vi "SeCrTs-Datalog Display NS creater.vi"(9 "Data FIFO Ref":T1) -> ()   [LabVIEW 2022 SP3]
uses:
  RT Controls/SeCrTs-Data FIFO.ctl
  RT Controls/SeCrTs-DiplayPC comm ctrl.ctl
  <vilib>/dex/Stream Element Allocation Mode.ctl
  SeCrTs-RT_Global_R.vi
  <resource>/objmgr/ni.dex.rc
panel:
  out "Numeric":i32
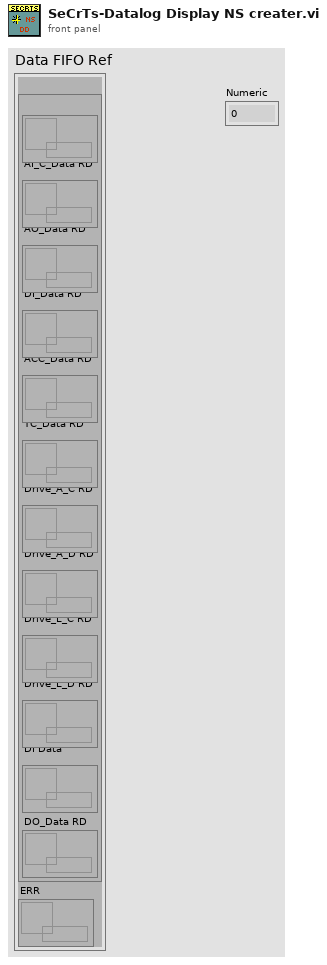
[diagram p1: front panel]
types:
  T1 = typedef "SeCrTs-Data FIFO.ctl" = cluster{"RD":cluster{"AI_V_Data RD":refnum<queue>, "AI_C_Data RD":refnum<queue>, "AO_Data RD":refnum<queue>, "DI_Data RD":refnum<queue>, "ACC_Data RD":refnum<queue>, "TC_Data RD":refnum<queue>, "Drive_A_C RD":refnum<queue>, "Drive_A_D RD":refnum<queue>, "Drive_L_C RD":refnum<queue>, "Drive_L_D RD":refnum<queue>, "DI Data":refnum<queue>, "DO_Data RD":refnum<queue>}, "ERR":refnum<queue>}
  T2 = typedef "SeCrTs-DiplayPC comm ctrl.ctl" = enum16{"Initialize", "Listen for UI Writer", "Send RT Data"}
  T3 = typedef "Stream Element Allocation Mode.ctl" = u32
  T4 = cluster{"Start DAQ":bool, "Stop DAQ":bool, "RT Stop":bool, "RT Exit":bool, "Start Seq":bool}
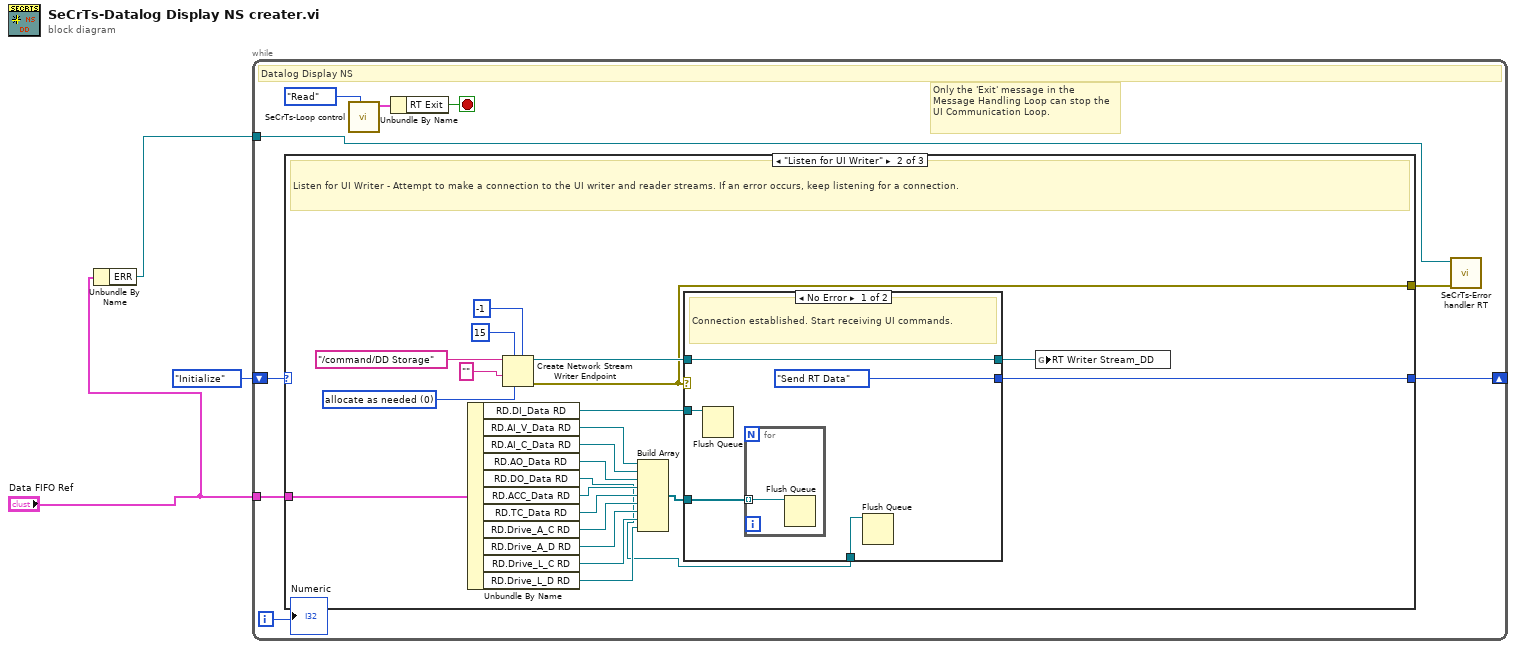
[diagram p0: block diagram]
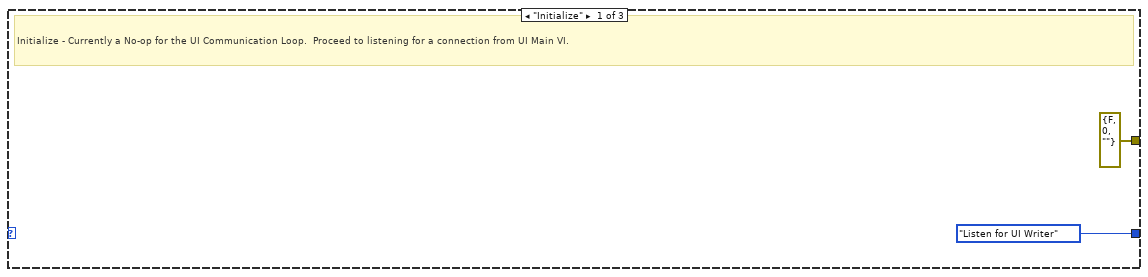
[diagram p2: hidden frame]
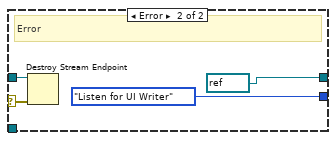
[diagram p3: hidden frame]
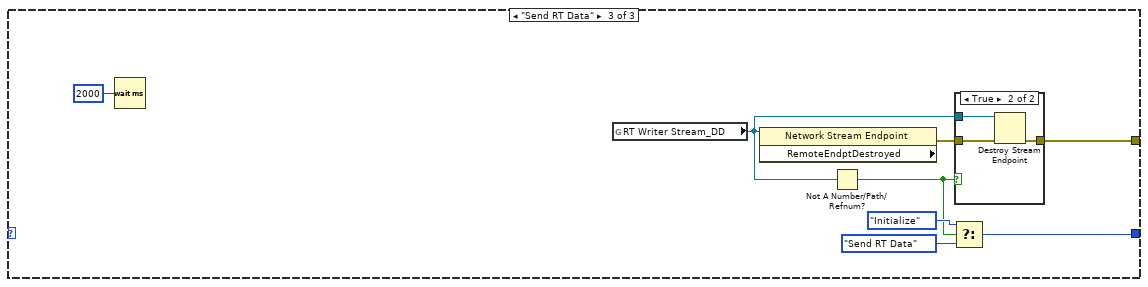
[diagram p4: hidden frame]
diagram:
  n1 = Unbundle By Name("Data FIFO Ref") -> ("ERR"=w1:refnum<queue>)
  n2 = while {
    shift-right: [w12] -> _
    shift-left: SeCrTs-DiplayPC_comm_ctrl."Initialize" -> [w11]
    tunnel: "Data FIFO Ref" -> [w10]
    tunnel: w1 -> [w6]
    i -> [w4]
    stop <- w7 stop-if-true
    # "Only the 'Exit' message in the  Message Handling Loop can stop the UI Communication Loop."
    # "Datalog Display NS"
    n3 = case shown="\"Listen for UI Writer\"" w11 {
      tunnel: [errorcluster {"status"=FALSE, "code"=0, "source"=""} ("error IO") w35 w47] -> w5
      tunnel: [SeCrTs-DiplayPC_comm_ctrl."Listen for UI Writer" w34 w53] -> w12
      tunnel: w10 -> [_ w31 _]
      frame "Initialize" {
        # "Initialize - Currently a No-op for the UI Communication Loop.  Proceed to listening for a connection from UI Main VI."
      }
      frame "Listen for UI Writer" {
        w16 = T3 0 items=["allocate as needed", "pre-allocate"] ("element allocation mode")
        # "Listen for UI Writer - Attempt to make a connection to the UI writer and reader streams. If an error occurs, keep listening for a connection."
        n4 = Unbundle By Name(w31) -> ("RD.DI_Data RD"=w18:refnum<queue>, "RD.AI_V_Data RD"=w28:refnum<queue>, "RD.AI_C_Data RD"=w27:refnum<queue>, "RD.AO_Data RD"=w26:refnum<queue>, "RD.DO_Data RD"=w15:refnum<queue>, "RD.ACC_Data RD"=w25:refnum<queue>, "RD.TC_Data RD"=w24:refnum<queue>, "RD.Drive_A_C RD"=w23:refnum<queue>, "RD.Drive_A_D RD"=w22:refnum<queue>, "RD.Drive_L_C RD"=w21:refnum<queue>, "RD.Drive_L_D RD"=w20:refnum<queue>)
        n5 = Create Network Stream Writer Endpoint(5:-1 ("timeout in ms (-1)"), 6:w16, 7:15 ("writer buffer size"), 9:"" ("reader url"), 11:"/command/DD Storage" ("reader url")) -> (0:w35:errorcluster, 3:w36:refnum<k21>)  [unwired: 2 in]
        n6 = Build Array(w28, w27, w26, w25, w24, w23, w22, w21, w20) -> (w19:refnum<queue>[])
        n7 = case shown="No Error" w35 {
          selector: w35 -> [_ w44]
          tunnel: w36 -> [w40 w46]
          tunnel: [SeCrTs-DiplayPC_comm_ctrl."Send RT Data" SeCrTs-DiplayPC_comm_ctrl."Listen for UI Writer"] -> w34
          tunnel: [w40 refnum<k21> refnum ("reader url")] -> w29
          tunnel: w19 -> [w39 _]
          tunnel: w18 -> [w38 _]
          tunnel: w15 -> [w37 _]
          frame No Error {
            # "Connection established. Start receiving UI commands."
            n8 = Flush Queue(queue=w38) -> ()  [unwired: 1 in, 3 out]
            n9 = for {
              tunnel: w39 -> [w42] mode=indexing
              n10 = Flush Queue(queue=w42) -> ()  [unwired: 1 in, 3 out]
            }
            n11 = Flush Queue(queue=w37) -> ()  [unwired: 1 in, 3 out]
          }
          frame Error {
            # "Error"
            n12 = Destroy Stream Endpoint(8:w44, 11:w46) -> ()  [unwired: 1 out]
          }
        }
        n13 = global write "SeCrTs-RT_Global_R.vi" "RT Writer Stream_DD"(w29) -> ()
      }
      frame "Send RT Data" {
        n14 = Wait (ms)(milliseconds to wait=u32 2000) -> ()  [unwired: 1 out]
        n15 = global read "SeCrTs-RT_Global_R.vi" "RT Writer Stream_DD"() -> (w49:refnum<k21>)
        n16 = property class="Network Stream Endpoint" props=["RemoteEndptDestroyed"](reference=w49) -> (error out=w48:errorcluster)  [unwired: 1 in, 2 out]
        n17 = Not A Number/Path/Refnum?(number/path/refnum=w49) -> (NaN/Path/Refnum?=w50:bool)
        n18 = Select(t=SeCrTs-DiplayPC_comm_ctrl."Initialize", s=w50, f=SeCrTs-DiplayPC_comm_ctrl."Send RT Data") -> (s? t:f=w53:T2)
        n19 = case shown="True" w50 {
          tunnel: w49 -> [_ w58]
          tunnel: w48 -> [w55 w57]
          tunnel: [w55 w56] -> w47
          frame False {
          }
          frame True {
            n20 = Destroy Stream Endpoint(8:w57, 11:w58) -> (0:w56:errorcluster)
          }
        }
      }
    }
    n21 = call "SeCrTs-Loop control.vi"("Action"=enum16{"Init", "Write", "Read"}."Read") -> ("Loop Control out"=w9:T4)  [unwired: 9 in, 1 out]
    n22 = Unbundle By Name(w9) -> ("RT Exit"=w7:bool)
    n23 = call "SeCrTs-Error handler RT.vi"("error in"=w5, "Message Queue"=w6) -> ()  [unwired: 8 in, 2 out]
    "Numeric" <- w4
  }
